vi "Acroname_Port_Disable.vi"(8 "error in (no error)":errorcluster, 11 "Port Number":i32) -> (0 "error out":errorcluster)   [LabVIEW 2025]
uses:
  1b1786e0-183b-4c19-b690-1d9e1fdb2131.vi
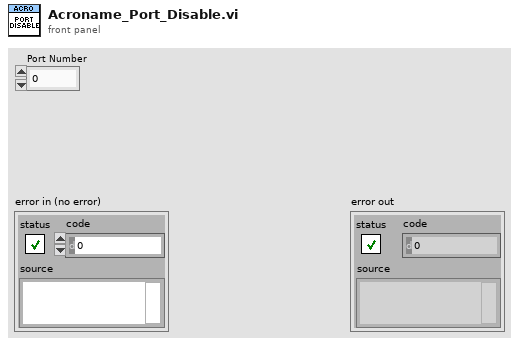
[diagram p1: front panel]
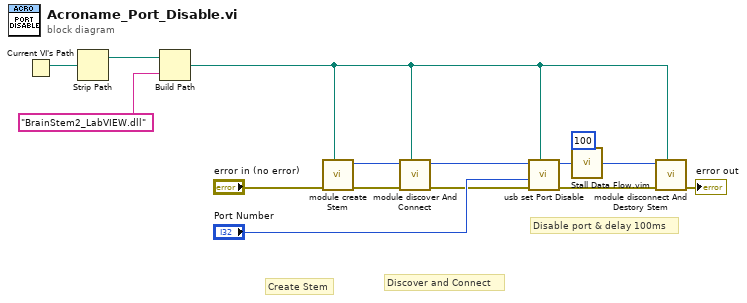
[diagram p0: block diagram]
diagram:
  # "Disable port & delay 100ms"
  # "Discover and Connect"
  # "Create Stem"
  n1 = Current VI's Path() -> (path=w4:path)
  n2 = Strip Path(path=w4) -> (stripped path=w3:path)  [unwired: 1 out]
  n3 = Build Path(base path=w3, name or relative path="BrainStem2_LabVIEW.dll") -> (appended path=w1:path)
  n4 = call "module create Stem.vi"("dll path in"=w1, "error in (no error)"="error in (no error)") -> ("error out"=w11:errorcluster, "id out"=w15:u32)  [unwired: 7 in, 1 out]
  n5 = call "module discover And Connect.vi"("dll path in"=w1, "error in (no error)"=w11, "id"=w15) -> ("error out"=w10:errorcluster, "id out"=w14:u32)  [unwired: 6 in, 1 out]
  n6 = call "usb set Port Disable.vi"("dll path in"=w1, "error in (no error)"=w10, "channel"="Port Number", "id"=w14) -> ("error out"=w8:errorcluster, "id out"=w6:u32)  [unwired: 5 in, 1 out]
  n7 = call "Stall Data Flow.vim"("value in"=w6, "milliseconds to wait"=100) -> ("value out"=w13:u32)  [unwired: 1 out]
  n8 = call "module disconnect And Destory Stem.vi"("dll path in"=w1, "error in (no error)"=w8, "id"=w13) -> ("error out"=→"error out":errorcluster)  [unwired: 6 in, 2 out]
